vi "RR autofocus view-calibrate.vi"() -> ()   [LabVIEW 2011]
uses:
  Autofocus Globals.vi
  Instance           1 35Saved   RR autofocus view-calibrate .vi
panel:
  out "Intensity 3":dbl(graph)
  out "Intensity 2":cluster{"X position":dbl, "Y position":dbl}(graph)
  out "Calibration curve":cluster{ext[], dbl[]}(graph)
  in  "Do calibration":bool
  out "Intensity":dbl(graph)
  out "XY Position":cluster{"Y":dbl[], "Y":dbl[]}[](graph)=[{"Y"=[30.68], "Y"=[27.36]}]
  in  "Quit":bool
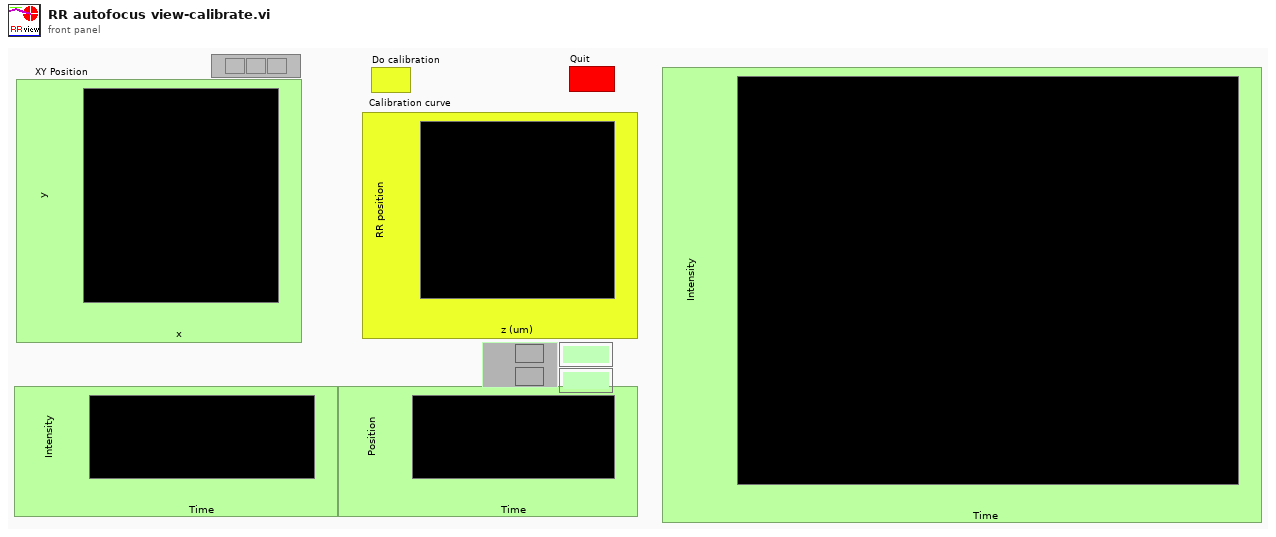
[diagram p1: front panel]
types:
  T1 = typedef "Laser type.ctt" = enum16{"Blue 488 nm", "Green 532 nm", "Orange 594 nm", "Red 633 nm", "IR 780"}
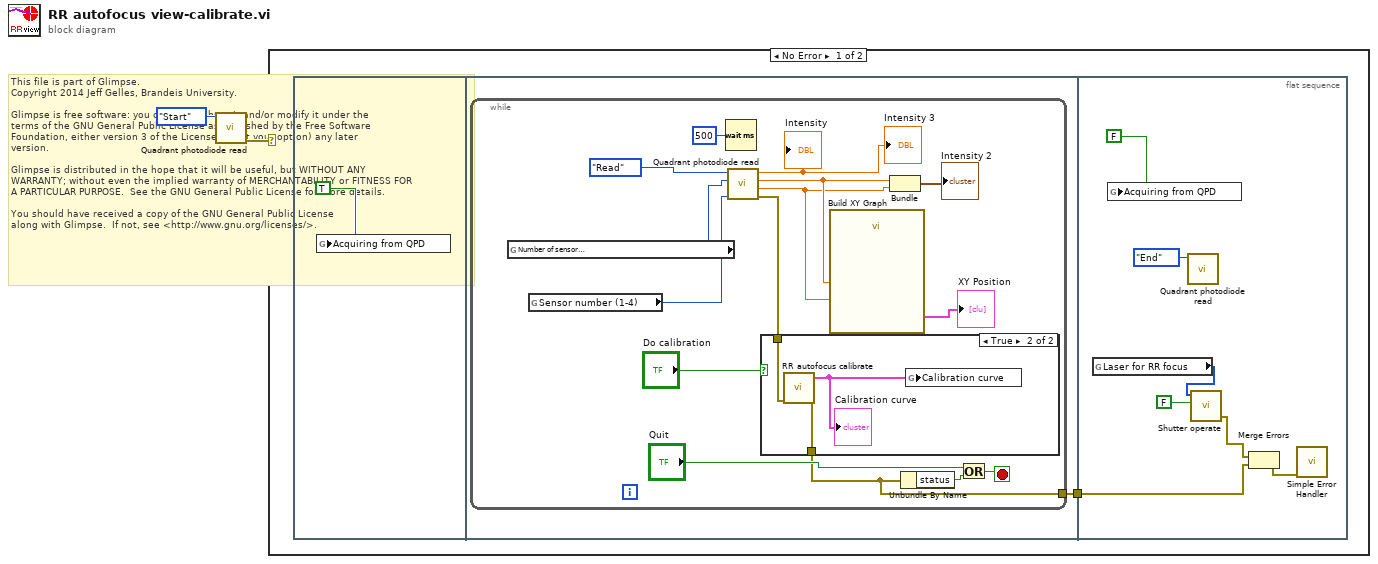
[diagram p0: block diagram]
diagram:
  # "This file is part of Glimpse. \nCopyright 2014 Jeff Gelles, Brandeis University.    \n\nGlimpse is free software: you can redistribute it and/or modify it under the \nterms of the GNU General Public License as published by the Free Software \nFoundation, either version 3 of the License, or (at your option) any later \nversion.\n\nGlimpse is distributed in the hope that it will be useful, but WITHOUT ANY \nWARRANTY; without even the implied warranty of MERCHANTABILITY or FITNESS FOR \nA PARTICULAR PURPOSE.  See the GNU General Public License for more details.\n\nYou should have received a copy of the GNU General Public License\nalong with Glimpse.  If not, see <http://www.gnu.org/licenses/>."
  n1 = call "Quadrant photodiode read.vi"("Mode"=enum16{"Start", "Read", "End"}."Start") -> ("error out"=w2:errorcluster)  [unwired: 2 in, 6 out]
  n2 = case shown="No Error" w2 {
    frame No Error {
      n3 = flat-sequence {
        tunnel: [w5] -> w3
        tunnel: w3 -> [w25]
        frame #0 {
          n4 = global write "Autofocus Globals.vi" "Acquiring from QPD"(TRUE ("Acquiring from QPD")) -> ()
        }
        frame #1 {
          n5 = while {
            tunnel: [w7] -> w5
            stop <- w16 stop-if-true
            n6 = global read "Autofocus Globals.vi" "Number of sensor\nreadings to average"() -> (w13:i32)
            n7 = global read "Autofocus Globals.vi" "Sensor number (1-4)"() -> (w14:i8)
            n8 = Wait (ms)(milliseconds to wait=u32 500) -> ()  [unwired: 1 out]
            n9 = call "Quadrant photodiode read.vi"("Sensor Number\n(ignored)"=w14, "number of readings\n to average"=w13, "Mode"=enum16{"Start", "Read", "End"}."Read") -> ("error out"=w11:errorcluster, "Y position"=w9:dbl, "X position"=w10:dbl, "Power"=→"Intensity" →"Intensity 3":dbl)  [unwired: 3 out]
            n10 = case shown="True" "Do calibration" {
              tunnel: w11 -> [w21 w24]
              tunnel: [w21 w23] -> w7
              frame False {
              }
              frame True {
                n11 = call "RR autofocus calibrate.vi"("error in"=w24) -> ("error out"=w23:errorcluster, "Cal. curve"=w22:cluster{ext[], dbl[]})  [unwired: 9 out]
                "Calibration curve" <- w22
                n12 = global write "Autofocus Globals.vi" "Calibration curve"(w22) -> ()
              }
            }
            n13 = call "Build XY Graph"("Y Input"=w9, "X Input"=w10) -> ("XY Graph"=→"XY Position":cluster{"Y":dbl[], "Y":dbl[]}[])  [unwired: 3 in, 6 out]
            n14 = Bundle("X position"=w10, "Y position"=w9) -> (→"Intensity 2":cluster{"X position":dbl, "Y position":dbl})  [unwired: 1 out]
            n15 = Unbundle By Name(w7) -> ("status"=w15:bool)
            n16 = Or(x="Quit", y=w15) -> (x .or. y?=w16:bool)
          }
        }
        frame #2 {
          n17 = global read "Autofocus Globals.vi" "Laser for RR focus"() -> (w28:T1[])
          n18 = global write "Autofocus Globals.vi" "Acquiring from QPD"(FALSE ("Acquiring from QPD")) -> ()
          n19 = call "Quadrant photodiode read.vi"("Mode"=enum16{"Start", "Read", "End"}."End") -> ()  [unwired: 2 in, 7 out]
          n20 = call "Shutter operate.vi"("Shutters"=w28, 2:FALSE ("Data to Write")) -> ("error out"=w26:errorcluster)  [unwired: 1 in, 5 out]
          n21 = Merge Errors(w26, w25) -> (w27:errorcluster)
          n22 = call <vilib>:"Simple Error Handler.vi"("error in (no error)"=w27) -> ()  [unwired: 1 in, 8 out]
        }
      }
    }
    frame Error {
      # "error"
    }
  }
